vi "Calc ScaleFactorNew.vi"(8 "error in (no error)":errorcluster, 11 "[A/D Input]":dbl[][](array[numeric])) -> (0 "error out":errorcluster, 1 "ScaleFactorB":i32, 2 "ScaleFactorA":i32, 3 "Pass?":bool, 4 "May Pass Retest?":bool, 5 "Test Results":dbl[][](array[numeric]) format="%.2f", 9 "Pass/Fail #":i32)   [LabVIEW 2013]
uses:
  InputScript states.ctl
  <vilib>/Utility/NIReport.llb/NI_report.lvclass
  <vilib>/addons/_office/excel.llb/Excel Easy Table (num).vi
  <vilib>/addons/_office/excel.llb/Excel Get Data ([str]).vi
  <vilib>/addons/_office/excel.llb/Excel Get Data ([dbl]).vi
  <vilib>/addons/_office/NI_ReportGenerationToolkit.lvlib
  <vilib>/Utility/NIReport.llb/Excel/NI_Excel.lvclass
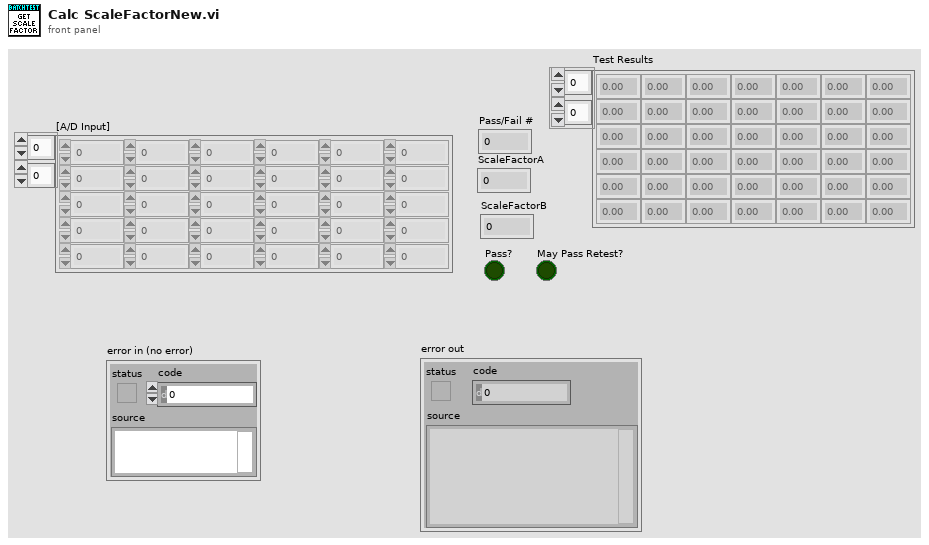
[diagram p1: front panel]
types:
  T1 = typedef "InputScript states.ctl" = enum16{"Open Template", "Write Values", "Read Results", "Close Template"}
  T2 = enum16{"maximized", "minimized", "normal", "no change"}
  T3 = enum16{"Standard Report", "HTML", "Word", "Excel"}
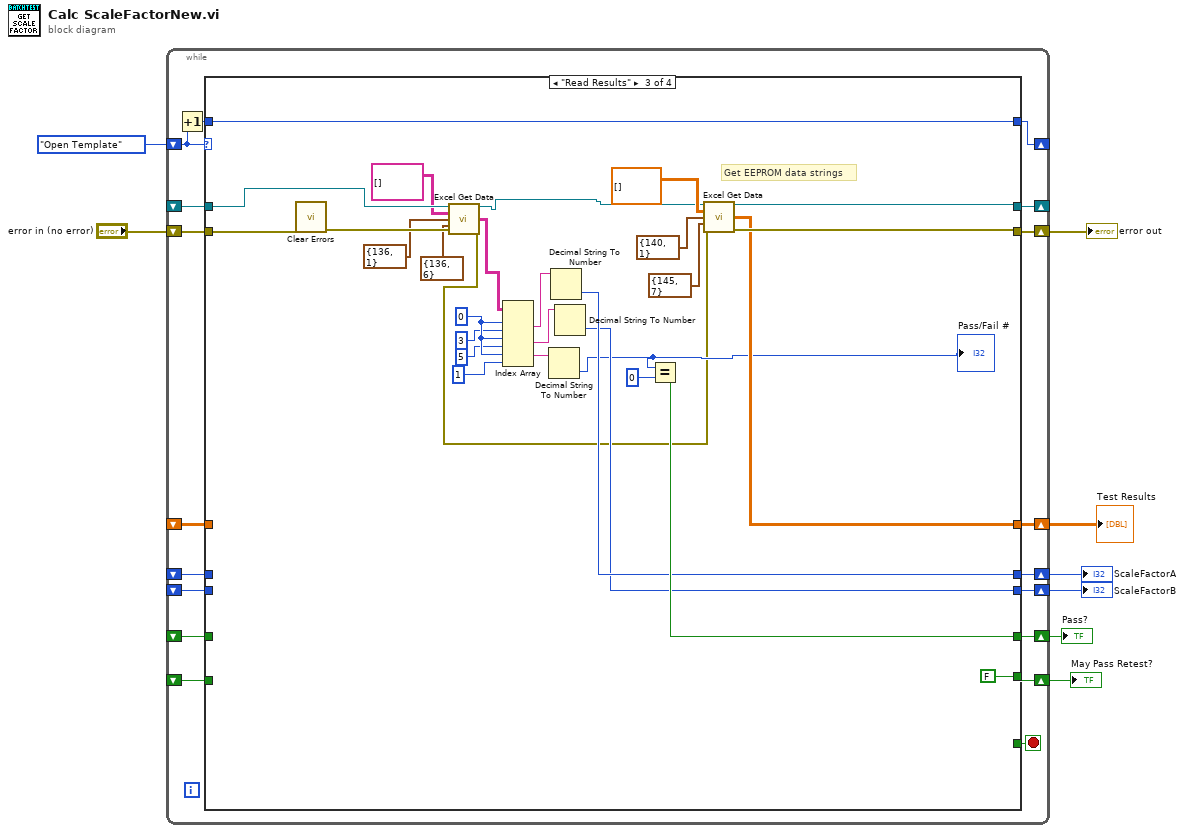
[diagram p0: block diagram]
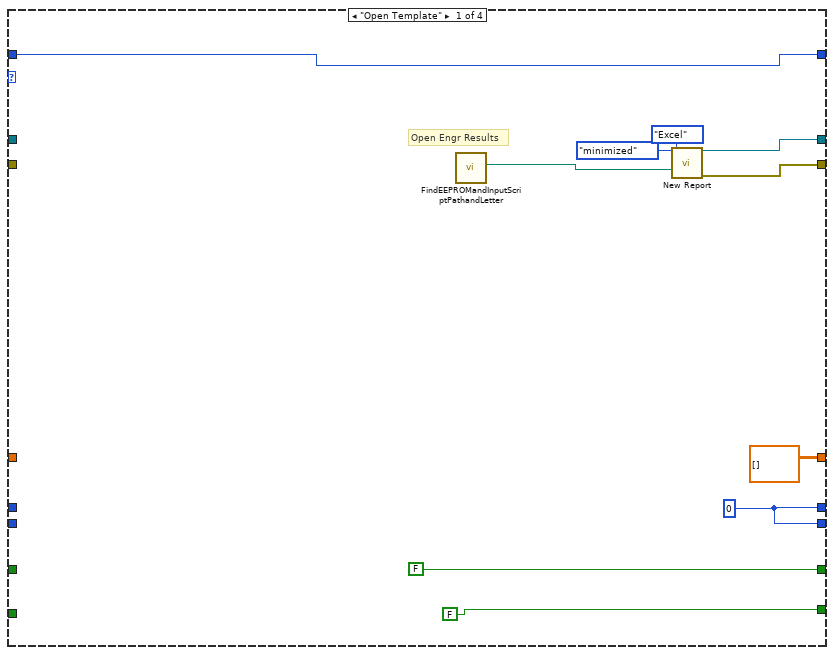
[diagram p2: hidden frame]
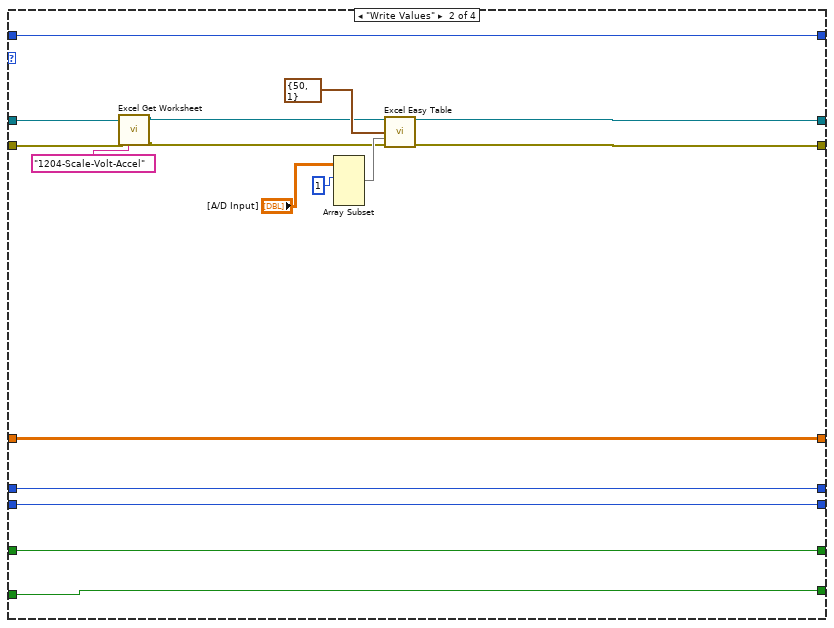
[diagram p3: hidden frame]
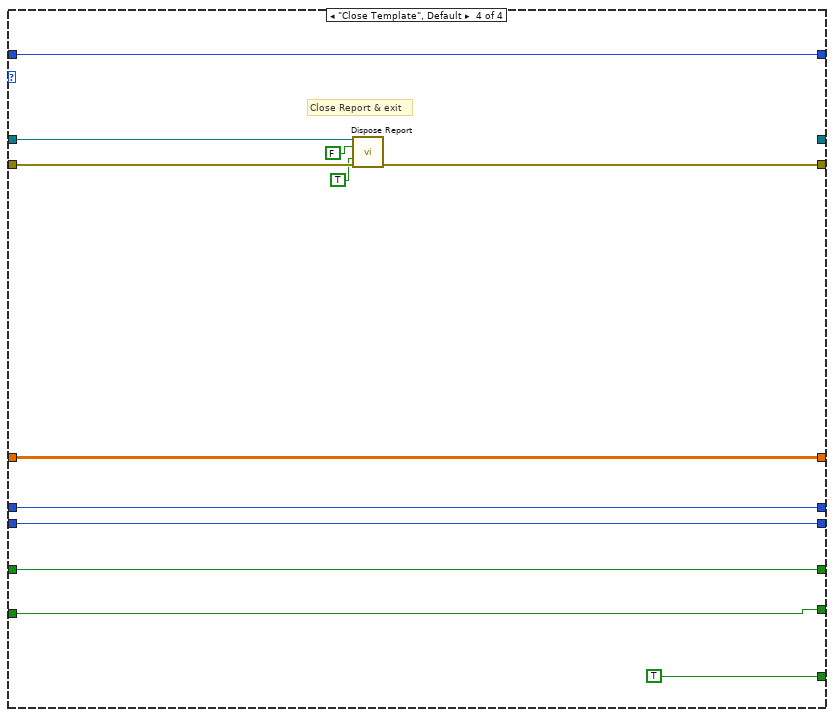
[diagram p4: hidden frame]
diagram:
  n1 = while {
    shift-right: [w25] -> _
    shift-left: _ -> [w24]
    shift-right: [w23] -> w6
    shift-left: "error in (no error)" -> [w22]
    shift-right: [w19] -> _
    shift-left: InputScript_states."Open Template" -> [w21]
    shift-right: [w18] -> w5
    shift-left: _ -> [w17]
    shift-right: [w16] -> w2
    shift-left: _ -> [w15]
    shift-right: [w14] -> w4
    shift-left: _ -> [w13]
    shift-right: [w12] -> w3
    shift-left: _ -> [w11]
    shift-right: [w10] -> w1
    shift-left: _ -> [w9]
    stop <- w26 stop-if-true
    n2 = Increment(x=w21) -> (x+1=w20:T1)
    n3 = case shown="\"Read Results\"" w21 {
      tunnel: [_ _ _ TRUE] -> w26
      tunnel: [w36 w48 w75 _] -> w25
      tunnel: w24 -> [_ w43 w73 w93]
      tunnel: [w35 w47 w77 w91] -> w23
      tunnel: w22 -> [_ w41 w72 w92]
      tunnel: w20 -> [w34 w53 w82 w89]
      tunnel: [w34 w53 w82 w89] -> w19
      tunnel: [w33 w52 w79 w88] -> w18
      tunnel: w17 -> [_ w52 _ w88]
      tunnel: [FALSE w50 w81 w87] -> w16
      tunnel: w15 -> [_ w50 _ w87]
      tunnel: [w33 w49 w78 w86] -> w14
      tunnel: w13 -> [_ w49 _ w86]
      tunnel: [FALSE w46 FALSE w84] -> w12
      tunnel: w11 -> [_ w46 _ w84]
      tunnel: [dbl[][] [] ("data") w38 w76 w83] -> w10
      tunnel: w9 -> [_ w38 _ w83]
      frame "Open Template" {
        w33 = u8 0 ("ScaleFactor")
        # "Open Engr Results"
        n4 = call "FindEEPROMandInputScriptPathandLetter.vi"() -> ("Engr Result Path"=w27:path)  [unwired: 7 in, 2 out]
        n5 = call <vilib>:"New Report.vi"("window state (normal)"=T2."minimized", "report type"=T3."Excel", "template (empty)"=w27) -> ("report out"=w36:refnum<class "NI_report.lvclass">, "error out"=w35:errorcluster)  [unwired: 11 in]
      }
      frame "Write Values" {
        n6 = call <vilib>:"Excel Get Worksheet.vi"("report in"=w43, "error in (no error)"=w41, "name (\"\")"="1204-Scale-Volt-Accel" ("name (\"\")")) -> ("report out"=w42:refnum<class "NI_report.lvclass">, "error out"=w40:errorcluster)  [unwired: 11 in]
        n7 = Array Subset(array="[A/D Input]", index (row)=1 ("length")) -> (w44:dbl[][])  [unwired: 3 in]
        n8 = call-poly <vilib>:"Excel Easy Table.vi"("report in"=w42, "start (0, 0)"=cluster{"row":i32, "column":i32} {"row"=50, "column"=1} ("start (-1, -1)"), "text data"=w44, "error in (no error)"=w40) -> ("report out"=w48:refnum<class "NI_report.lvclass">, "error out"=w47:errorcluster)  [unwired: 7 in, 3 out]
      }
      frame "Read Results" {
        w68 = 0 ("index (row)")
        # "Get EEPROM data strings"
        n9 = call <vilib>:"Clear Errors.vi"("error in (no error)"=w72) -> ("error out"=w71:errorcluster)  [unwired: 6 in]
        n10 = call-poly <vilib>:"Excel Get Data.vi"("report in"=w73, "data type"=string[][] [], "start (-1, -1)"=cluster{"row":i32, "column":i32} {"row"=136, "column"=1}, "end (-1, -1)"=cluster{"row":i32, "column":i32} {"row"=136, "column"=6}, "error in (no error)"=w71) -> ("report out"=w54:refnum<class "NI_report.lvclass">, "data"=w60:string[][], "error out"=w55:errorcluster)  [unwired: 8 in]
        n11 = Index Array(array=w60, index (row) #1=w68, index (col) #1=3 ("disabled index (col)"), index (row) #2=w68, index (col) #2=5 ("disabled index (col)"), index (row) #3=w68, index (col) #3=1 ("disabled index (col)")) -> (element #1=w63:string, element #2=w62:string, element #3=w61:string)
        n12 = Decimal String To Number(string=w61) -> (number=w74:i32)  [unwired: 2 in, 1 out]
        "Pass/Fail #" <- w74
        n13 = Decimal String To Number(string=w63) -> (number=w79:i32)  [unwired: 2 in, 1 out]
        n14 = Decimal String To Number(string=w62) -> (number=w78:i32)  [unwired: 2 in, 1 out]
        n15 = Equal?(x=w74, y=0) -> (x = y?=w81:bool)
        n16 = call-poly <vilib>:"Excel Get Data.vi"("report in"=w54, "data type"=dbl[][] [], "start (-1, -1)"=cluster{"row":i32, "column":i32} {"row"=140, "column"=1}, "end (-1, -1)"=cluster{"row":i32, "column":i32} {"row"=145, "column"=7}, "error in (no error)"=w55) -> ("report out"=w75:refnum<class "NI_report.lvclass">, "data"=w76:dbl[][], "error out"=w77:errorcluster)  [unwired: 8 in]
      }
      frame "Close Template", Default {
        # "Close Report & exit"
        n17 = call-dynamic "Dispose Report.vi"("report in"=w93, "wait until printing completed? (T)"=FALSE, "save changes? (F)"=TRUE, "error in (no error)"=w92) -> ("error out"=w91:errorcluster)  [unwired: 11 in]
      }
    }
  }
  "error out" <- w6
  "ScaleFactorA" <- w5
  "Pass?" <- w2
  "ScaleFactorB" <- w4
  "May Pass Retest?" <- w3
  "Test Results" <- w1
